vi "AI_Core_r1.vi"(10 "InitializeAI?":bool, 11 "AI_Pin_Cluster":T1={"CONV"="RMC/DIO0", "RST"="RMC/DIO64", "SCK"="RMC/DIO17", "CS"="RMC/DIO81", "BUSY"="RMC/DIO16", "DOUT_A"="RMC/DIO48", "DOUT_B"="RMC/DIO80", "t_RST (ticks)"=0, "t_CONV (ticks)"=0, "t_BUSYMAX (ticks)"=0}) -> (2 "8Ch_Data[]":i16[](array[numeric]))   [LabVIEW 2018, in "AI_FPGA.lvlib"]
uses:
  AI_FPGA.lvlib
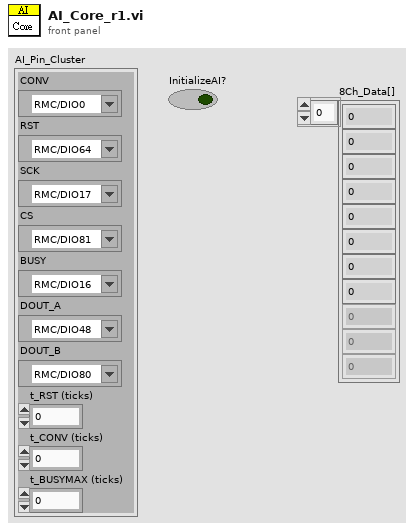
[diagram p1: front panel]
types:
  T1 = cluster{"CONV":refnum<k21>, "RST":refnum<k21>, "SCK":refnum<k21>, "CS":refnum<k21>, "BUSY":refnum<k21>, "DOUT_A":refnum<k21>, "DOUT_B":refnum<k21>, "t_RST (ticks)":u32, "t_CONV (ticks)":u32, "t_BUSYMAX (ticks)":u32}
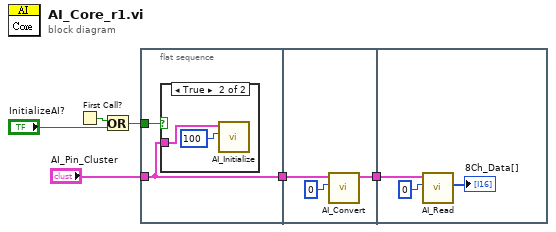
[diagram p0: block diagram]
diagram:
  n1 = First Call?() -> (First Call?: T/F=w6:bool)
  n2 = Or(x=w6, y="InitializeAI?") -> (x .or. y?=w4:bool)
  n3 = flat-sequence {
    tunnel: w4 -> [w8]
    tunnel: "AI_Pin_Cluster" -> [w7]
    tunnel: [w7] -> w2
    tunnel: w2 -> [w12]
    tunnel: [w11] -> w1
    tunnel: w1 -> [w14]
    frame #0 {
      n4 = case shown="True" w8 {
        tunnel: w7 -> [_ w9]
        frame False {
        }
        frame True {
          n5 = call "AI_Initialize.vi"("t_RST (ticks)"=u32 100, "AD7606_IO in"=w9) -> ()  [unwired: 9 in, 1 out]
        }
      }
    }
    frame #1 {
      n6 = call "AI_Convert.vi"("t_CONV (ticks)"=u32 0, "AD7606_IO in"=w12) -> ("AD7606_IO out"=w11:T1)  [unwired: 9 in]
    }
    frame #2 {
      n7 = call "AI_Read.vi"("t_CLK (ticks)"=u32 0, "AD7606_IO in"=w14) -> ("Data[]"=→"8Ch_Data[]":i16[])  [unwired: 8 in, 1 out]
    }
  }
